vi "Directional Speed 1.0 In Place Input Write Structure.vi"(5 "Device Inputs":dbl[](array[numeric]), 7 "Last Device Inputs":dbl[](array[numeric]), 8 "error in (no error)":errorcluster, 9 "FPGA ref in":T1, 11 "1.0 Directional Speed in":T2) -> (0 "error out":errorcluster, 1 "FPGA ref out":T1, 3 "1.0 Directional Speed out":T2)   [LabVIEW 2013, in "Engine Simulation Toolkit Engine.lvlib"]
uses:
  Engine Simulation Toolkit Engine.lvlib
  Shared/1.0 Directional Speed Engine Data.ctl
  Shared/1.0 Directional Speed FIFO Idxs.ctl
  Directional Speed 1.0 Input Ref.ctl
  Directional Speed 1.0 FPGA Inputs Write Node.vi
  Shared/Engine Simulation Toolkit Shared.lvlib
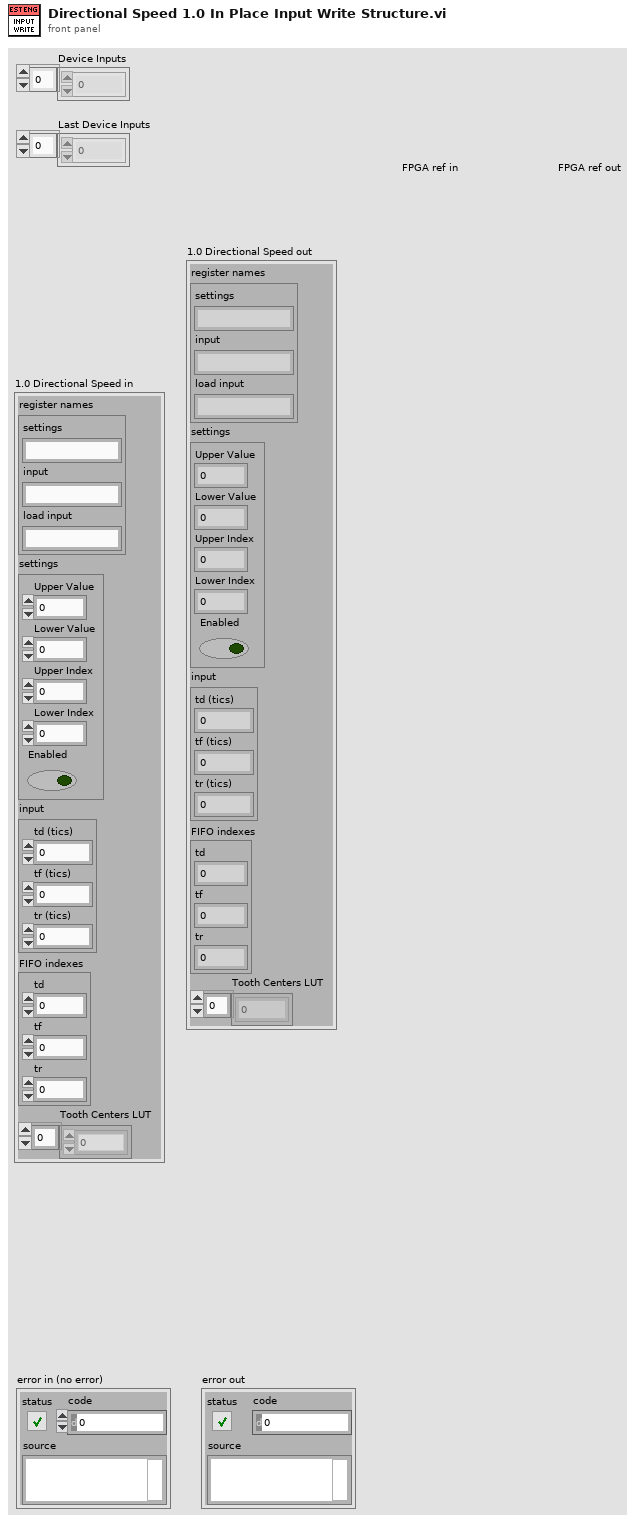
[diagram p1: front panel]
types:
  T1 = typedef "Engine Simulation Toolkit Engine.lvlib/Directional Speed 1.0 Input Ref.ctl" = refnum<k20>
  T2 = typedef "Engine Simulation Toolkit Shared.lvlib/1.0 Directional Speed Engine Data.ctl" = cluster{"register names":cluster{"settings":string, "input":string, "load input":string}, "settings":cluster{"Upper Value":u16, "Lower Value":u16, "Upper Index":fxp<+,10,10>, "Lower Index":fxp<+,10,10>, "Enabled":bool}, "input":cluster{"td (tics)":u16, "tf (tics)":u16, "tr (tics)":u16}, "FIFO indexes":T3, "Tooth Centers LUT":u16[]}
  T3 = typedef "Engine Simulation Toolkit Shared.lvlib/1.0 Directional Speed FIFO Idxs.ctl" = cluster{"td":i32, "tf":i32, "tr":i32}
  T4 = cluster{"td (tics)":u16, "tf (tics)":u16, "tr (tics)":u16}
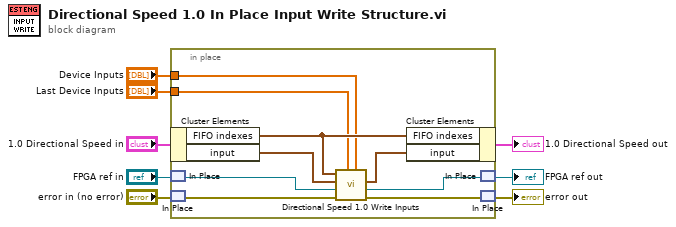
[diagram p0: block diagram]
diagram:
  n1 = in-place {
    in-place-border: "Last Device Inputs" -> [w12]
    in-place-border: "Device Inputs" -> [w11]
    n2 = in-place-cluster #1("1.0 Directional Speed in") -> ("FIFO indexes"=w14:T3, "input"=w15:T4)
    n3 = in-place-match #2("FPGA ref in") -> (w10:T1)
    n4 = in-place-match #3("error in (no error)") -> (w17:errorcluster)
    n5 = call "Directional Speed 1.0 Write Inputs.vi"("Device inputs"=w11, "Last Device inputs"=w12, "error in (no error)"=w17, "input reference in"=w10, "input in"=w15, "FIFO indexes.inputs"=w14) -> ("error out"=w16:errorcluster, "input reference out"=w9:T1, "input out"=w13:T4)  [unwired: 3 in]
    n6 = in-place-cluster #1("FIFO indexes"=w14, "input"=w13) -> (→"1.0 Directional Speed out":T2)
    n7 = in-place-match #2(w9) -> (→"FPGA ref out":T1)
    n8 = in-place-match #3(w16) -> (→"error out":errorcluster)
  }
